vi "Control Value To Registry.vi"(4 "Registry Variant Accessor (optional)":refnum<class "CConfig Variant Accessor.lvclass">, 6 "Controls":refnum<vi>[](array[refnum]), 7 "Registry Control Reference Accessor (optional)":refnum<class "Registry Ctrl Ref Accessor.lvclass">, 8 "error in (no error)":errorcluster, 9 "Create keys? [T]":bool=TRUE, 10 "Create sections? [T]":bool=TRUE, 11 "Registry Object in":refnum<class "Carya Config.lvclass">) -> (0 "error out":errorcluster, 1 "Created key?":bool, 2 "Created session?":bool, 3 "Registry Object out":refnum<class "Carya Config.lvclass">, 5 "Used controls":refnum<vi>[](array[refnum]))   [LabVIEW 2013, in "Carya Config.lvclass"]
doc: "Copyright 2018, Carya Automatisering, Wiebe Walstra."
uses:
  Carya Config.lvclass
  CConfig Ctrl Ref Accessor/Registry Ctrl Ref Accessor.lvclass
  CConfig Variant Accessor/CConfig Variant Accessor.lvclass
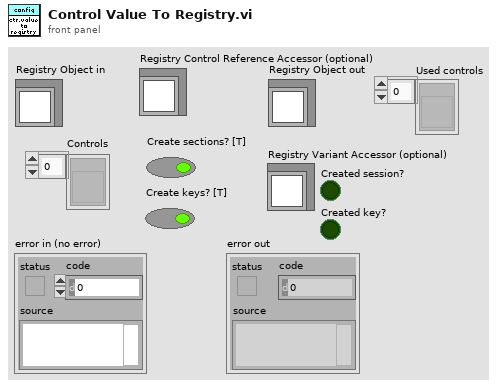
[diagram p1: front panel]
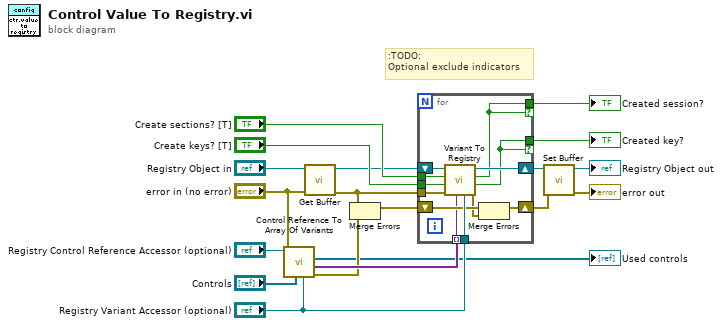
[diagram p0: block diagram]
diagram:
  # ":TODO:\nOptional exclude indicators"
  n1 = call-dynamic "Control Reference To Array Of Variants.vi"("Registry Variant Accessor"="Registry Variant Accessor (optional)", "Controls"="Controls", "error in (no error)"="error in (no error)", "Registry Control Reference Accessor in"="Registry Control Reference Accessor (optional)") -> ("error out"=w3:errorcluster, "Variants"=w9:variant[], "Controls"=→"Used controls":refnum<vi>[])  [unwired: 4 in, 1 out]
  n2 = call-dynamic "Get Buffer.vi"("error in (no error)"="error in (no error)", "Carya Config in"="Registry Object in") -> ("error out"=w11:errorcluster, "Config"=w5:refnum<class "Carya Config.lvclass">)  [unwired: 8 in]
  n3 = Merge Errors(w11, w3) -> (w4:errorcluster)
  n4 = for {
    tunnel: "Create sections? [T]" -> [w31]
    tunnel: "Create keys? [T]" -> [w30]
    tunnel: w11 -> [w29]
    tunnel: "Registry Variant Accessor (optional)" -> [w27]
    shift-right: [w26] -> w6
    shift-left: w5 -> [w28]
    shift-right: [w23] -> w10
    shift-left: w4 -> [w25]
    tunnel: w9 -> [w22] mode=indexing
    tunnel: [w21] -> w8 if=w21
    tunnel: [w20] -> w7 if=w20
    n5 = call "Variant To Registry.vi"("Registry Variant Accessor in"=w27, "Variant"=w22, "error in (no error)"=w29, "Create keys? [T]"=w30, "Create sections? [T]"=w31, "Carya Config in"=w28) -> ("error out"=w24:errorcluster, "Created key?"=w20:bool, "Created session?"=w21:bool, "Carya Config out"=w26:refnum<class "Carya Config.lvclass">)  [unwired: 2 in]
    n6 = Merge Errors(w25, w24) -> (w23:errorcluster)
  }
  "Created session?" <- w8
  "Created key?" <- w7
  n7 = call-dynamic "Set Buffer.vi"("error in (no error)"=w10, "Carya Config"=w6) -> ("error out"=→"error out":errorcluster, "Carya Config out"=→"Registry Object out":refnum<class "Carya Config.lvclass">)  [unwired: 8 in]
